vi "Abort Stream.vi"(0 "niUsrpRio Session":T1={"FPGA Interface"=refnum, "RIO Interface Number"=0, "Data Clock Rate"=0, "FPGA Data Clock Rate"=0, "Global Settings Register Bus"=refnum, "Radio 0 Settings Register Bus"=refnum, "Radio 1 Settings Register Bus"=refnum, "Radio Settings Bus Semaphore"=refnum, "DB Queues"=[], "Characterization Data Valid?"=FALSE, "EEPROM Header"={"Checksum"=0, "Product Code"=0, "Hardware Current Version"=0, "Hardware Oldest Compatible Version"=0, "EEPROM Map Current Version"=0, "EEPROM Map Oldest Compatible Version"=0, "User Password"="", "Pointer to Factory Header"=0, "Pointer to User Header"=0, "Recommended Interval"=0, "Number of Reserved Bytes"=9, "Number of Daughterboards"=0, "Daughterboard IDs"=[], "Daughterboard Serial Numbers"=[]}, "Device Data Header"={"Checksum"=0, "Number of Channels"=0, "Number of Gain Settings"=[], "Pointer to Characterization Data"=[], "Number of Reserved Bytes"=27, "Number of Frequencies"=[]}, "EEPROM Characterization Header"={"Checksum"=0, "Date"=timestamp(0 s since 1904-01-01), "Temperature"=0.0, "Misc. Info"="", "Pointer to Device Data Header"=0, "Number of Reserved Bytes"=28}, "Characterization Data"=[], "FPGA Current Version"=0, "FPGA Oldest Compatible Version"=0, "Fixed Logic Current Version"=0, "Fixed Logic Oldest Compatible Version"=0, "FPGA Radio Settings Bus Current Version"=0, "FPGA Radio Settings Bus Oldest Compatible Version"=0, "FPGA Board Config Current Version"=0, "FPGA Board Config Oldest Compatible Version"=0, "Daughterboard Clock Rate"=0, "daughterboard configuration session handles"=[]} {"Daughterboard Clock Rate" format="%#.3pHz"; "FPGA Data Clock Rate" format="%#.3pHz"; "Data Clock Rate" format="%#.3pHz"; "Characterization Data"."Frequencies [Hz]" format="%#_6p"; "EEPROM Characterization Header"."Pointer to Device Data Header" format="%x"; "EEPROM Characterization Header"."Checksum" format="%x"; "Device Data Header"."Pointer to Characterization Data" format="%x"; "Device Data Header"."Checksum" format="%x"; "EEPROM Header"."Pointer to User Header" format="%x"; "EEPROM Header"."Pointer to Factory Header" format="%x"; "EEPROM Header"."Product Code" format="%x"; "EEPROM Header"."Checksum" format="%x"}, 1 "scope":string(combo)="rx", 5 "check stream status":bool, 9 "timeout":dbl=10.0 format="%#_gs", 11 "error in":errorcluster) -> (4 "niUsrpRio Session (out)":T1={"FPGA Interface"=refnum, "RIO Interface Number"=0, "Data Clock Rate"=0, "FPGA Data Clock Rate"=0, "Global Settings Register Bus"=refnum, "Radio 0 Settings Register Bus"=refnum, "Radio 1 Settings Register Bus"=refnum, "Radio Settings Bus Semaphore"=refnum, "DB Queues"=[], "Characterization Data Valid?"=FALSE, "EEPROM Header"={"Checksum"=0, "Product Code"=0, "Hardware Current Version"=0, "Hardware Oldest Compatible Version"=0, "EEPROM Map Current Version"=0, "EEPROM Map Oldest Compatible Version"=0, "User Password"="", "Pointer to Factory Header"=0, "Pointer to User Header"=0, "Recommended Interval"=0, "Number of Reserved Bytes"=9, "Number of Daughterboards"=0, "Daughterboard IDs"=[], "Daughterboard Serial Numbers"=[]}, "Device Data Header"={"Checksum"=0, "Number of Channels"=0, "Number of Gain Settings"=[], "Pointer to Characterization Data"=[], "Number of Reserved Bytes"=27, "Number of Frequencies"=[]}, "EEPROM Characterization Header"={"Checksum"=0, "Date"=timestamp(0 s since 1904-01-01), "Temperature"=0.0, "Misc. Info"="", "Pointer to Device Data Header"=0, "Number of Reserved Bytes"=28}, "Characterization Data"=[], "FPGA Current Version"=0, "FPGA Oldest Compatible Version"=0, "Fixed Logic Current Version"=0, "Fixed Logic Oldest Compatible Version"=0, "FPGA Radio Settings Bus Current Version"=0, "FPGA Radio Settings Bus Oldest Compatible Version"=0, "FPGA Board Config Current Version"=0, "FPGA Board Config Oldest Compatible Version"=0, "Daughterboard Clock Rate"=0, "daughterboard configuration session handles"=[]} {"Daughterboard Clock Rate" format="%#.3pHz"; "FPGA Data Clock Rate" format="%#.3pHz"; "Data Clock Rate" format="%#.3pHz"; "Characterization Data"."Frequencies [Hz]" format="%#_6p"; "EEPROM Characterization Header"."Pointer to Device Data Header" format="%x"; "EEPROM Characterization Header"."Checksum" format="%x"; "Device Data Header"."Pointer to Characterization Data" format="%x"; "Device Data Header"."Checksum" format="%x"; "EEPROM Header"."Pointer to User Header" format="%x"; "EEPROM Header"."Pointer to Factory Header" format="%x"; "EEPROM Header"."Product Code" format="%x"; "EEPROM Header"."Checksum" format="%x"}, 15 "error out":errorcluster)   [LabVIEW 2018]
doc: "Aborts the acquisition/generation (based on the <b>scope</b> parameter), Waits for the stream to go idle, and then checks the stream status."
uses:
  FPGA/SubVIs/Stream Control State.ctl
  <instrlib>/niUsrpRio/Config/v1/Host/Public/niUsrpRio Session.ctl
  <instrlib>/_niInstr/Register Bus/v0/Host/Public/Register Bus Session.ctl
  <instrlib>/_niInstr/Register Bus/v0/Host/Private/Session Data.ctl
  <instrlib>/niUsrpRio/Config/v1/Host/Private/DB Queue Reference.ctl
  <instrlib>/niUsrpRio/Config/v1/Host/Private/Daughterboard Data.ctl
  <instrlib>/niUsrpRio/Config/v1/Host/Private/ATR state data.ctl
  <instrlib>/niUsrpRio/Config/v1/Host/Private/Antenna Configuration.ctl
  <instrlib>/niUsrpRio/Config/v1/Host/Private/CPLD Power Mode.ctl
  <instrlib>/niUsrpRio/Config/v1/Host/Public/EEPROM Header.ctl
  <instrlib>/niUsrpRio/Config/v1/Host/Public/EEPROM Device Data Header.ctl
  <instrlib>/niUsrpRio/Config/v1/Host/Public/EEPROM Characterization Header.ctl
  <instrlib>/niUsrpRio/Config/v1/Host/Public/Characterization Data.ctl
  <instrlib>/niUsrpRio/Config/v1/Host/Public/IQ Imbalance.ctl
  Streaming Xvcr FPGA Ref.ctl
  <vilib>/rvi/errors/niLvFpgaAdjustHostInterfaceError.vi
  <vilib>/rvi/interface/nirviReadWriteControl/nirviReadWriteControl.xnode
  <vilib>/rvi/interface/Simulation/niFpgaSimulationCallBeginRW.vi
  NiFpgaLv.dll
  <instrlib>/niUsrpRio/Config/v1/Host/niUsrpRio Config v1 Host.lvlib
  <instrlib>/_niInstr/Register Bus/v0/Host/niInstr Register Bus v0 Host.lvlib
panel:
  out "samples processed":u32
  out "state":T10
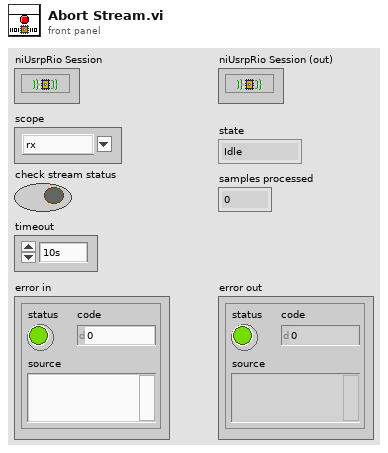
[diagram p1: front panel]
types:
  T1 = typedef "niUsrpRio Config v1 Host.lvlib/niUsrpRio Session.ctl" = cluster{"FPGA Interface":refnum<k20>, "RIO Interface Number":u32, "Data Clock Rate":u32, "FPGA Data Clock Rate":u32, "Global Settings Register Bus":T2, "Radio 0 Settings Register Bus":T2, "Radio 1 Settings Register Bus":T2, "Radio Settings Bus Semaphore":T3, "DB Queues":T4[], "Characterization Data Valid?":bool, "EEPROM Header":T5, "Device Data Header":T6, "EEPROM Characterization Header":T7, "Characterization Data":T8[], "FPGA Current Version":u32, "FPGA Oldest Compatible Version":u32, "Fixed Logic Current Version":u32, "Fixed Logic Oldest Compatible Version":u32, "FPGA Radio Settings Bus Current Version":u32, "FPGA Radio Settings Bus Oldest Compatible Version":u32, "FPGA Board Config Current Version":u32, "FPGA Board Config Oldest Compatible Version":u32, "Daughterboard Clock Rate":u32, "daughterboard configuration session handles":u64[]}
  T2 = typedef "niInstr Register Bus v0 Host.lvlib/Register Bus Session.ctl" = refnum<queue>
  T3 = typedef "Semaphore RefNum" = refnum<k1>
  T4 = typedef "niUsrpRio Config v1 Host.lvlib/DB Queue Reference.ctl" = refnum<queue>
  T5 = typedef "niUsrpRio Config v1 Host.lvlib/EEPROM Header.ctl" = cluster{"Checksum":u32, "Product Code":u16, "Hardware Current Version":u16, "Hardware Oldest Compatible Version":u16, "EEPROM Map Current Version":u16, "EEPROM Map Oldest Compatible Version":u16, "User Password":string, "Pointer to Factory Header":u32, "Pointer to User Header":u32, "Recommended Interval":u16, "Number of Reserved Bytes":i32, "Number of Daughterboards":u8, "Daughterboard IDs":u16[], "Daughterboard Serial Numbers":string[]}
  T6 = typedef "niUsrpRio Config v1 Host.lvlib/EEPROM Device Data Header.ctl" = cluster{"Checksum":u32, "Number of Channels":u8, "Number of Gain Settings":u16[], "Pointer to Characterization Data":u32[], "Number of Reserved Bytes":i32, "Number of Frequencies":u16[]}
  T7 = typedef "niUsrpRio Config v1 Host.lvlib/EEPROM Characterization Header.ctl" = cluster{"Checksum":u32, "Date":timestamp, "Temperature":sgl, "Misc. Info":string, "Pointer to Device Data Header":u32, "Number of Reserved Bytes":i32}
  T8 = typedef "niUsrpRio Config v1 Host.lvlib/Characterization Data.ctl" = cluster{"Gains[dB]":dbl[], "Frequencies [Hz]":dbl[], "IQ Imbalance Table":T9[], "Measured Gains[dB]":dbl[][]}
  T9 = typedef "niUsrpRio Config v1 Host.lvlib/IQ Imbalance.ctl" = cluster{"Gain Imbalance [linear]":dbl, "Phase Imbalance [radians]":dbl, "Offset":cdb}
  T10 = typedef "Stream Control State.ctl" = enum16{"Idle", "Active"}
  T11 = typedef "Streaming Xvcr FPGA Ref.ctl" = refnum<k20>
  T12 = typedef "niUsrpRio Config v1 Host.lvlib/Device Subfunction.ctl" = enum16{"rx", "tx", "all"}
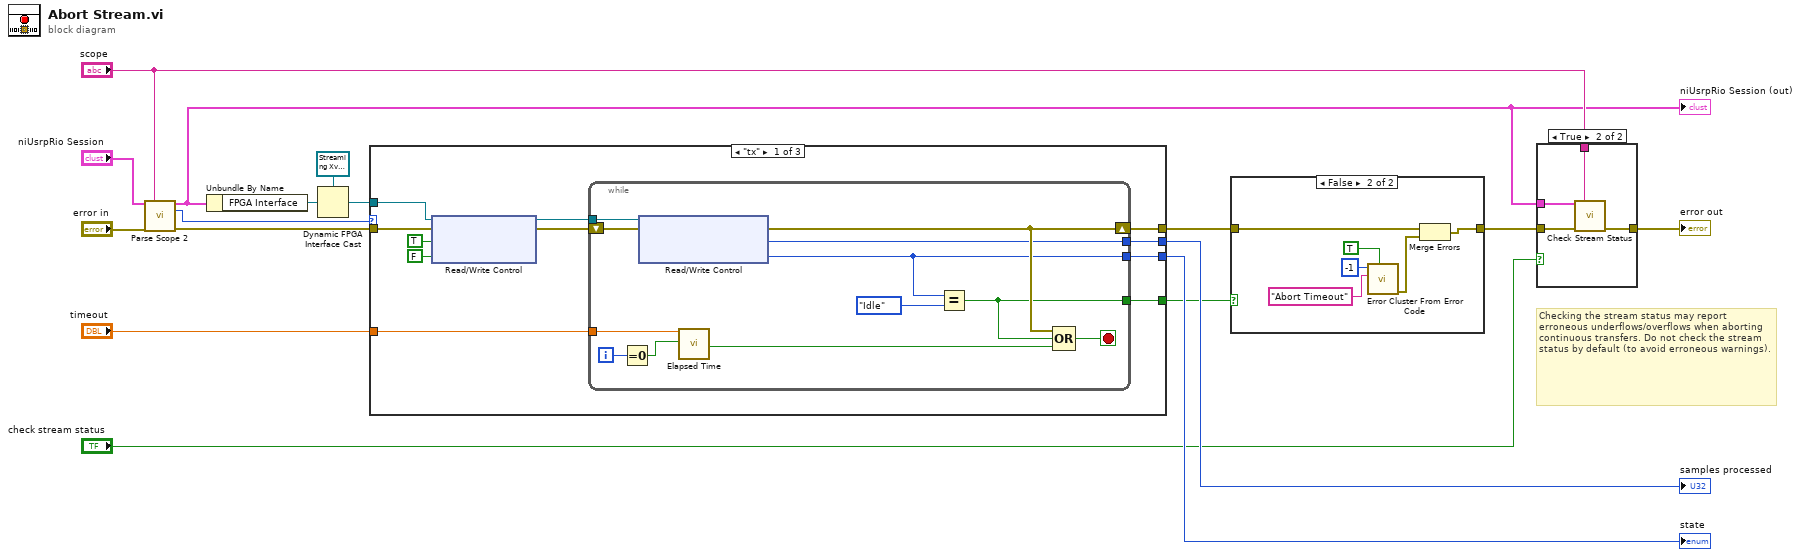
[diagram p0: block diagram]
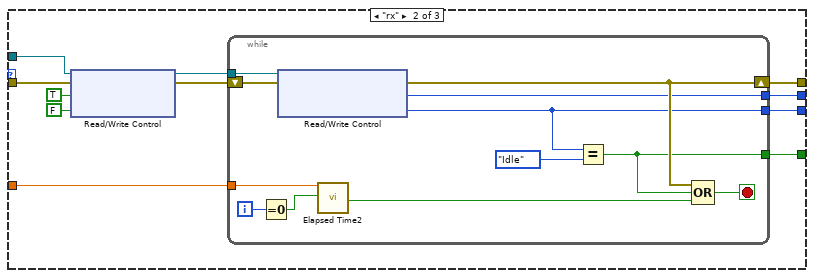
[diagram p3: hidden frame]
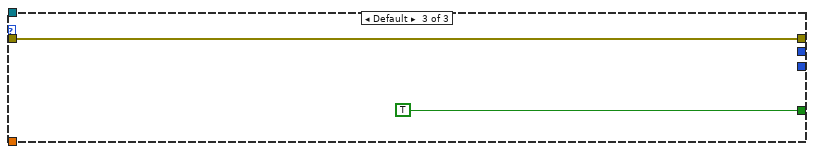
[diagram p4: hidden frame]
diagram:
  # "Checking the stream status may report erroneous underflows/overflows when aborting continuous transfers. Do not check the stream status by default (to avoid erroneous warnings)."
  n1 = call <instrlib>:"Parse Scope 2.vi"("niUsrpRio Session"="niUsrpRio Session", "scope"="scope", "error in"="error in") -> ("niUsrpRio Session (out)"=w2:T1, "Device Subfunction"=w8:T12, "error out"=w7:errorcluster)  [unwired: 4 in, 6 out]
  "niUsrpRio Session (out)" <- w2
  n2 = Unbundle By Name(w2) -> ("FPGA Interface"=w5:refnum<k20>)
  n3 = Dynamic FPGA Interface Cast(Session In=T11 refnum ("Type"), Type=w5) -> (Session Out=w4:T11)
  n4 = case shown="\"tx\"" w8 {
    tunnel: w7 -> [w28 w51 w65]
    tunnel: [w26 w49 w65] -> w17
    tunnel: [w23 w46 _] -> w16
    tunnel: [w22 w45 TRUE] -> w3
    tunnel: "timeout" -> [w21 w44 _]
    tunnel: [w20 w43 _] -> w14
    tunnel: w4 -> [w18 w41 _]
    frame "tx" {
      n5 = xnode "Read/Write Control"("FPGA VIリファレンス入力"=w18, "エラー入力"=w28, "tx.abort"=TRUE ("Tx.Reset"), "tx.trigger enable"=FALSE ("tx.enable trigger")) -> ("FPGA VIリファレンス出力"=w25:T11, "エラー出力"=w24:errorcluster)
      n6 = while {
        tunnel: w25 -> [w39]
        tunnel: [w34] -> w22
        shift-right: [w40] -> w26
        shift-left: w24 -> [w38]
        tunnel: [w31] -> w23
        tunnel: w21 -> [w30]
        tunnel: [w29] -> w20
        i -> [w36]
        stop <- w35 stop-if-true
        n7 = Equal To 0?(x=w36) -> (x = 0?=w37:bool)
        n8 = xnode "Read/Write Control"("FPGA VIリファレンス入力"=w39, "エラー入力"=w38) -> ("エラー出力"=w40:errorcluster, "tx.samples processed"=w29:u32, "tx.state"=w31:enum16{"Idle", "Active"})  [unwired: 1 out]
        n9 = call "Elapsed Time"("Time Target (s)"=w30, "Reset"=w37) -> ("Time has Elapsed"=w32:bool)  [unwired: 10 in, 7 out]
        n10 = Equal?(x=w31, y=Stream_Control_State."Idle" ("state")) -> (x = y?=w34:bool)
        n11 = Compound Arithmetic op=OR(w40, w34, w32) -> (w35:bool)
      }
    }
    frame "rx" {
      n12 = xnode "Read/Write Control"("FPGA VIリファレンス入力"=w41, "エラー入力"=w51, "rx.abort"=TRUE ("Tx.Reset"), "rx.trigger enable"=FALSE ("rx.enable trigger")) -> ("FPGA VIリファレンス出力"=w48:T11, "エラー出力"=w47:errorcluster)
      n13 = while {
        tunnel: w48 -> [w62]
        tunnel: [w57] -> w45
        shift-right: [w63] -> w49
        shift-left: w47 -> [w61]
        tunnel: [w54] -> w46
        tunnel: w44 -> [w53]
        tunnel: [w52] -> w43
        i -> [w59]
        stop <- w58 stop-if-true
        n14 = Equal To 0?(x=w59) -> (x = 0?=w60:bool)
        n15 = xnode "Read/Write Control"("FPGA VIリファレンス入力"=w62, "エラー入力"=w61) -> ("エラー出力"=w63:errorcluster, "rx.samples processed"=w52:u32, "rx.state"=w54:enum16{"Idle", "Active"})  [unwired: 1 out]
        n16 = call "Elapsed Time2"("Time Target (s)"=w53, "Reset"=w60) -> ("Time has Elapsed"=w55:bool)  [unwired: 10 in, 7 out]
        n17 = Equal?(x=w54, y=Stream_Control_State."Idle" ("state")) -> (x = y?=w57:bool)
        n18 = Compound Arithmetic op=OR(w63, w57, w55) -> (w58:bool)
      }
    }
    frame Default {
    }
  }
  "state" <- w16
  "samples processed" <- w14
  n19 = case shown="FALSE" w3 {
    tunnel: w17 -> [w66 w71]
    tunnel: [w66 w69] -> w13
    frame True {
    }
    frame False {
      n20 = call <vilib>:"Error Cluster From Error Code.vi"("show call chain? (False)"=TRUE, "error message (\"\")"="Abort Timeout" ("error message (\"\")"), "error code (0)"=-1) -> ("error out"=w70:errorcluster)  [unwired: 6 in]
      n21 = Merge Errors(w71, w70) -> (w69:errorcluster)
    }
  }
  n22 = case shown="TRUE" "check stream status" {
    tunnel: w13 -> [w73 w77]
    tunnel: [w73 w76] -> w12
    tunnel: w2 -> [_ w75]
    tunnel: "scope" -> [_ w74]
    frame False {
    }
    frame True {
      n23 = call "Check Stream Status.vi"("niUsrpRio Session"=w75, "scope"=w74, "error in"=w77) -> ("error out"=w76:errorcluster)  [unwired: 10 in, 2 out]
    }
  }
  "error out" <- w12
